vi "MessageName.vi"() -> (2 "MessageName":string)   [LabVIEW 2020, in "SyncTicks.lvlib"]
uses:
  SyncTicks.lvlib
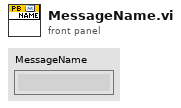
[diagram p1: front panel]
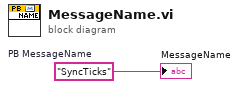
[diagram p0: block diagram]
diagram:
  w1 = "SyncTicks"  # PB MessageName
  "MessageName" <- w1
